vi "Configure Timebase.vi"(8 "error in (no error)":errorcluster, 9 "Time Delay (0.0 s)":dbl, 10 "Timebase (1E-6 s)":dbl=1e-06, 11 "VISA resource name":refnum<visa-resource-name>) -> (0 "error out":errorcluster, 3 "VISA resource name out":refnum<visa-resource-name>)   [LabVIEW 2011, in "Agilent DSO1000 Series.lvlib"]
doc: "Configures the timebase and horizontal features of the oscilloscope."
uses:
  <instrlib>/Agilent DSO1000 Series/Agilent DSO1000 Series.lvlib
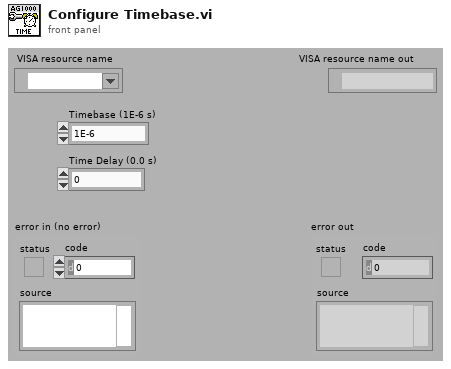
[diagram p1: front panel]
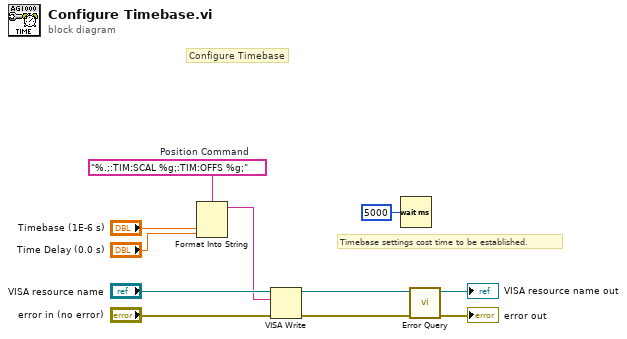
[diagram p0: block diagram]
diagram:
  w7 = "%.;:TIM:SCAL %g;:TIM:OFFS %g;"  # Position Command
  # "Timebase settings cost time to be established."
  # "Configure Timebase"
  n1 = Format Into String(format string=w7, "Timebase (1E-6 s)", "Time Delay (0.0 s)") -> (resulting string=w6:string)  [unwired: 2 in, 1 out]
  n2 = VISA Write(VISA resource name="VISA resource name", write buffer=w6, error in (no error)="error in (no error)") -> (VISA resource name out=w3:refnum<visa-resource-name>, error out=w2:errorcluster)  [unwired: 1 out]
  n3 = Wait (ms)(milliseconds to wait=u32 5000) -> ()  [unwired: 1 out]
  n4 = call <instrlib>:"Error Query.vi"("error in (no error)"=w2, "VISA resource name"=w3) -> ("error out"=→"error out":errorcluster, "VISA resource name out"=→"VISA resource name out":refnum<visa-resource-name>)  [unwired: 6 in, 2 out]
